vi "NIMS_dfd_Convert Band Specs (Lpth Norm).vi"(8 "W":dbl[](array[numeric]), 9 "Amplitude":dbl[](array[numeric]), 10 "Edges":dbl[](array[numeric]), 11 "F":dbl[](array[numeric])) -> (0 "error out":errorcluster, 2 "band specs":T1(array[cluster])=[{"frequency point"=[{"frequency"=0.0, "magnitude"=1.0, "weight"=1.0, "phase"=0.0}, {"frequency"=0.2, "magnitude"=1.0, "weight"=1.0, "phase"=0.0}]}, {"frequency point"=[{"frequency"=0.3, "magnitude"=0.0, "weight"=1.0, "phase"=0.0}, {"frequency"=0.5, "magnitude"=0.0, "weight"=1.0, "phase"=0.0}]}] {"frequency point"."weight" format="%.2f"})   [LabVIEW 2017, in "NI_DigFilter_MathScript.lvlib"]
uses:
  <vilib>/addons/Digital Filter Design/NI_DigFilter_MathScript.lvlib
  <vilib>/addons/Digital Filter Design/_Misc.llb/dfd_Error Handlers (Multiple).vi
  <vilib>/addons/Digital Filter Design/NI_DigFilterLicensed.lvlib
panel:
  # "freq"
  # "magnitude"
  # "weight"
  # "phase"
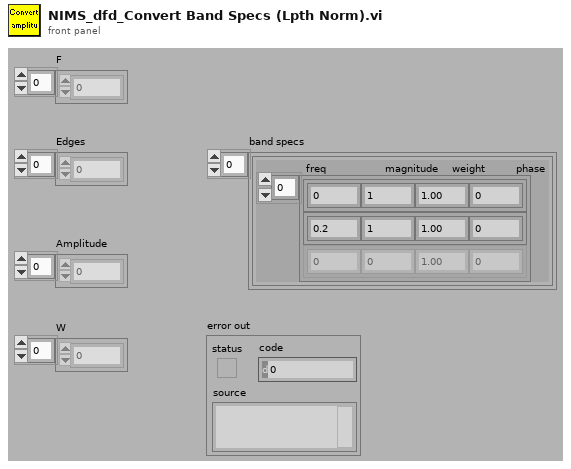
[diagram p1: front panel]
types:
  T1 = cluster{"frequency point":cluster{"frequency":dbl, "magnitude":dbl, "weight":dbl, "phase":dbl}[]}[]
  T2 = cluster{"Numeric":dbl, "Numeric":dbl, "Numeric":dbl, dbl}
  T3 = cluster{cluster{"Numeric":dbl, "Numeric":dbl, "Numeric":dbl, dbl}[]}
  T4 = cluster{cluster{"Numeric":dbl, "Numeric":dbl, dbl, dbl}[]}
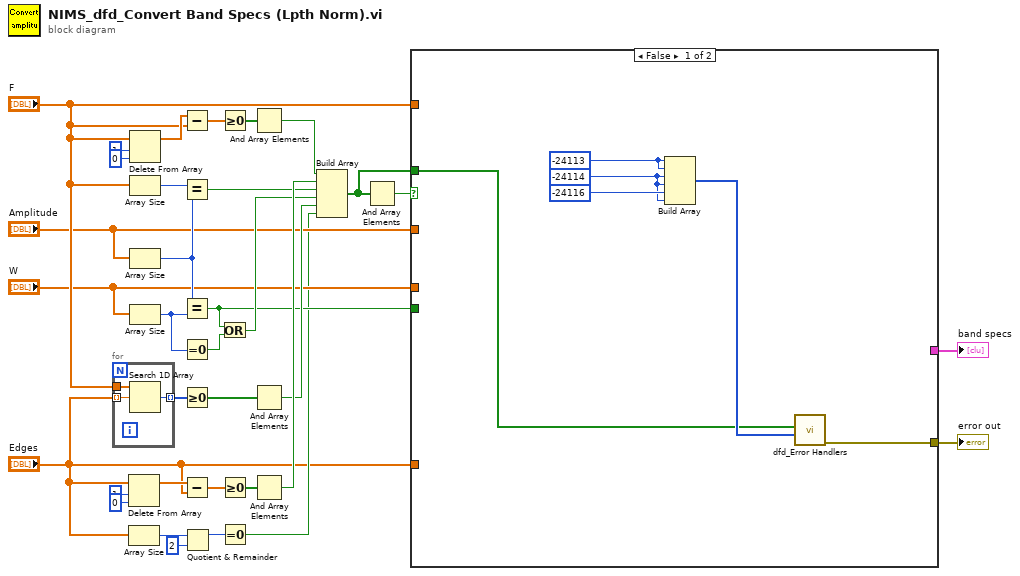
[diagram p0: block diagram]
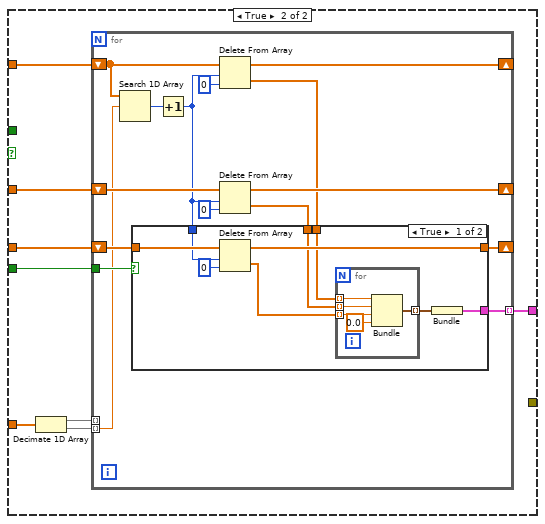
[diagram p2: hidden frame]
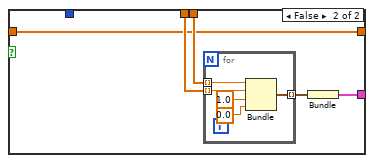
[diagram p3: hidden frame]
diagram:
  n1 = for {
    tunnel: "F" -> [w37]
    tunnel: "Edges" -> [w36] mode=indexing
    tunnel: [w35] -> w19 mode=indexing
    n2 = Search 1D Array(1D array=w37, element=w36) -> (index of element=w35:i32)  [unwired: 1 out]
  }
  n3 = Delete From Array(array="Edges", length=1, index=0) -> (array with subset deleted=w13:dbl[])  [unwired: 1 out]
  n4 = Array Size(array="Edges") -> (size(s)=w8:i32)
  n5 = Delete From Array(array="F", length=1, index=0) -> (array with subset deleted=w32:dbl[])  [unwired: 1 out]
  n6 = Array Size(array="F") -> (size(s)=w26:i32)
  n7 = Array Size(array="Amplitude") -> (size(s)=w25:i32)
  n8 = Array Size(array="W") -> (size(s)=w24:i32)
  n9 = Subtract(x=w32, y="F") -> (x-y=w31:dbl[])
  n10 = Equal?(x=w26, y=w25) -> (x = y?=w21:bool)
  n11 = Equal?(x=w25, y=w24) -> (x = y?=w10:bool)
  n12 = Equal To 0?(x=w24) -> (x = 0?=w11:bool)
  n13 = Greater Or Equal To 0?(x=w19) -> (x >= 0?=w18:bool[])
  n14 = Subtract(x=w13, y="Edges") -> (x-y=w28:dbl[])
  n15 = Quotient & Remainder(x=w8, y=2) -> (x-y*floor(x/y)=w6:i32)  [unwired: 1 out]
  n16 = Greater Or Equal To 0?(x=w31) -> (x >= 0?=w30:bool[])
  n17 = Or(x=w10, y=w11) -> (x .or. y?=w20:bool)
  n18 = Greater Or Equal To 0?(x=w28) -> (x >= 0?=w29:bool[])
  n19 = Equal To 0?(x=w6) -> (x = 0?=w5:bool)
  n20 = And Array Elements(Boolean array=w30) -> (logical AND=w23:bool)
  n21 = And Array Elements(Boolean array=w18) -> (logical AND=w17:bool)
  n22 = And Array Elements(Boolean array=w29) -> (logical AND=w22:bool)
  n23 = Build Array(w23, w22, w21, w20, w17, w5) -> (w1:bool[])
  n24 = And Array Elements(Boolean array=w1) -> (logical AND=w2:bool)
  n25 = case shown="False" w2 {
    tunnel: "F" -> [_ w50]
    tunnel: "Amplitude" -> [_ w49]
    tunnel: "W" -> [_ w48]
    tunnel: "Edges" -> [_ w51]
    tunnel: [_ w47] -> w3
    tunnel: [w39 _] -> w12
    tunnel: w10 -> [_ w46]
    tunnel: w1 -> [w38 _]
    frame False {
      w40 = -24114 ("element")
      w42 = -24113
      n26 = Build Array(w42, w42, w40, w40, -24116 ("element"), w40) -> (w43:i32[])
      n27 = call-poly <vilib>:"dfd_Error Handlers.vi"("error sources"=w43, "condition failed?"=w38) -> ("error out"=w39:errorcluster)  [unwired: 1 in, 8 out]
    }
    frame True {
      n28 = Decimate 1D Array(w51) -> (w45:dbl[], w44:dbl[])
      n29 = for {
        tunnel: w45 -> [_] mode=indexing
        shift-right: [w63] -> _
        shift-left: w50 -> [w66]
        shift-right: [w58] -> _
        shift-left: w49 -> [w61]
        shift-right: [w57] -> _
        shift-left: w48 -> [w60]
        tunnel: [w54] -> w47 mode=indexing
        tunnel: w46 -> [w53]
        tunnel: w44 -> [w52] mode=indexing
        n30 = Search 1D Array(1D array=w66, element=w52) -> (index of element=w64:i32)  [unwired: 1 out]
        n31 = Increment(x=w64) -> (x+1=w59:i32)
        n32 = Delete From Array(array=w66, length=w59, index=0) -> (deleted portion=w56:dbl[], array with subset deleted=w63:dbl[])
        n33 = Delete From Array(array=w61, length=w59, index=0) -> (deleted portion=w55:dbl[], array with subset deleted=w58:dbl[])
        n34 = case shown="True" w53 {
          tunnel: w60 -> [w74 w81]
          tunnel: w59 -> [w73 _]
          tunnel: [w72 w81] -> w57
          tunnel: w56 -> [w71 w85]
          tunnel: w55 -> [w70 w84]
          tunnel: [w67 w82] -> w54
          frame True {
            n35 = Delete From Array(array=w74, length=w73, index=0) -> (deleted portion=w69:dbl[], array with subset deleted=w72:dbl[])
            n36 = for {
              tunnel: w71 -> [w80] mode=indexing
              tunnel: w70 -> [w79] mode=indexing
              tunnel: w69 -> [w78] mode=indexing
              tunnel: [w77] -> w68 mode=indexing
              n37 = Bundle("Numeric"=w80, "Numeric"=w79, "Numeric"=w78, 0.0) -> (w77:T2)  [unwired: 1 out]
            }
            n38 = Bundle(w68) -> (w67:T3)  [unwired: 1 in]
          }
          frame False {
            n39 = for {
              tunnel: w85 -> [w90] mode=indexing
              tunnel: w84 -> [w89] mode=indexing
              tunnel: [w88] -> w83 mode=indexing
              n40 = Bundle("Numeric"=w90, "Numeric"=w89, 1.0, 0.0) -> (w88:cluster{"Numeric":dbl, "Numeric":dbl, dbl, dbl})  [unwired: 1 out]
            }
            n41 = Bundle(w83) -> (w82:T4)  [unwired: 1 in]
          }
        }
      }
    }
  }
  "error out" <- w12
  "band specs" <- w3
